vi "solar QTimers Launch.vi"(6 "Suppress Errors? (T)":bool=TRUE, 8 "error in (no error)":errorcluster, 10 "Default QTimers":T1[](array[typedef]), 11 "solar in":refnum<class "solar.lvclass">) -> (0 "error out":errorcluster, 3 "solar out":refnum<class "solar.lvclass">)   [LabVIEW 2018]
doc: "This loads the QTimers from the target's configuration file.\nQTimers = \"TEST1,TEST2\"\nQTimer_TEST1 = \"1000,false,IgnoreIfExists\" # Test 1 QTimer EnQ's every second\nQTimer_TEST1_Msgs = \"READ{bool:true,dbl:3.14}\"\nQTimer_TEST2 = \"5000\" # Test 2 QTimer EnQ's every 5 seconds\nQTimer_TEST2_Msgs = \"READ{bool:true,dbl:3.14}\""
uses:
  qtimer/solar_qtimer_ctl QTimer Settings.ctl
  cfg/solar_cfg Read File (Str).vi
  solar.lvclass
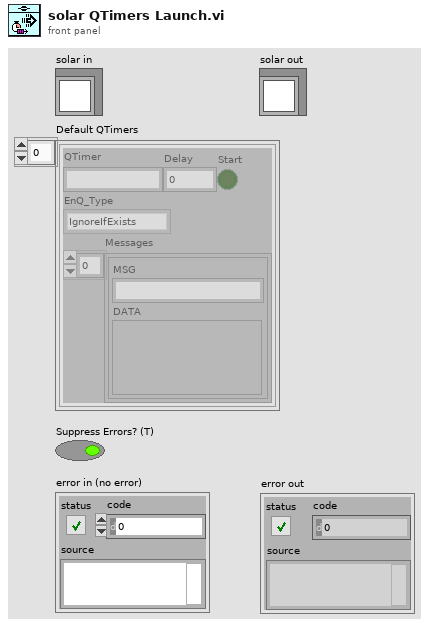
[diagram p1: front panel]
types:
  T1 = typedef "solar_qtimer_ctl QTimer Settings.ctl" = cluster{"QTimer":string, "Delay":i32, "Start":bool, "EnQ_Type":enum8{"Normal", "Priority", "IgnoreIfExists"}, "Messages":cluster{"MSG":string, "DATA":variant}[]}
  T2 = typedef "solar_qtimer_ctl Refnum.ctl" = refnum<k1>
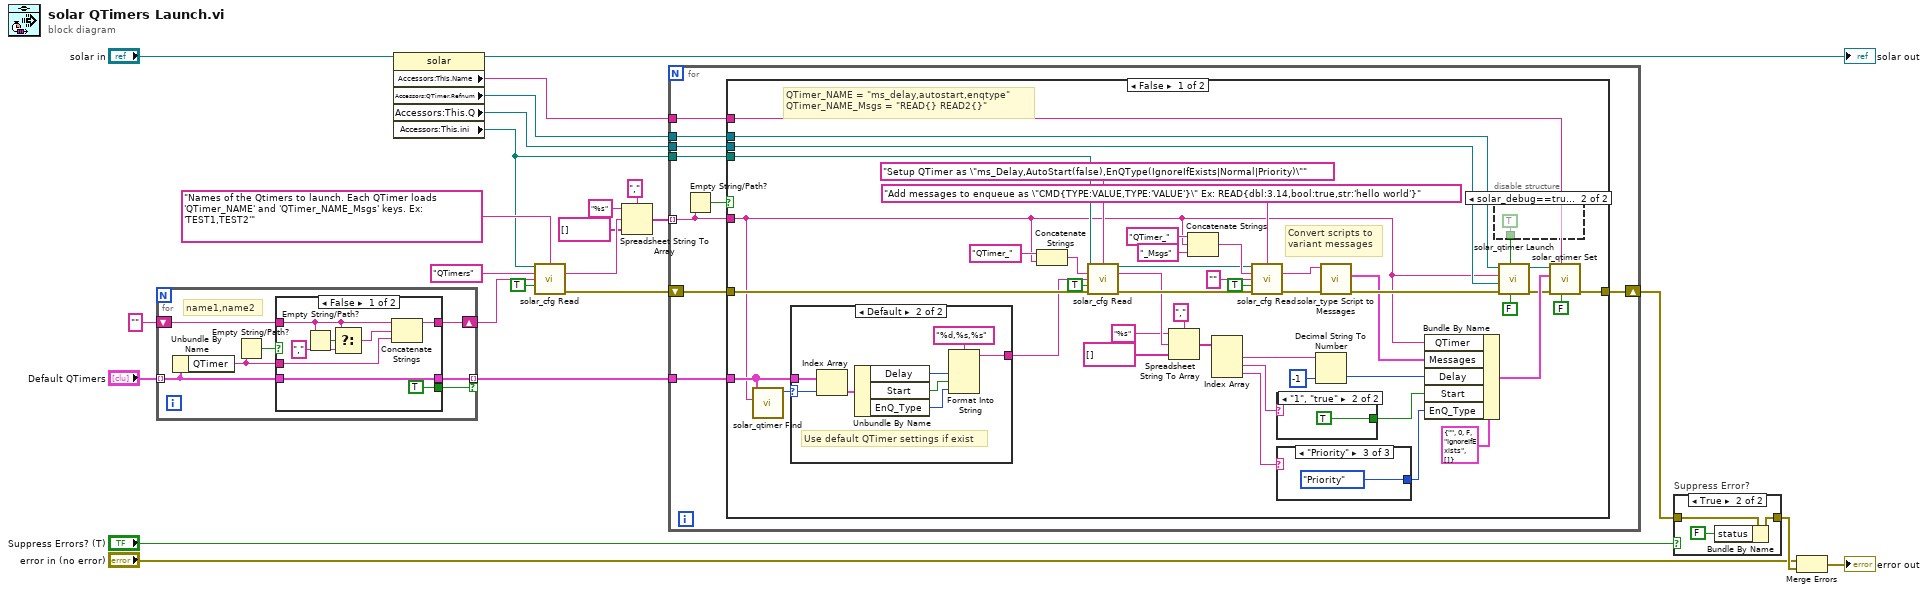
[diagram p0: block diagram]
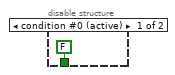
[diagram p2: hidden frame]
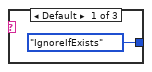
[diagram p3: hidden frame]
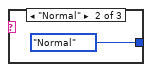
[diagram p4: hidden frame]
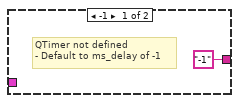
[diagram p6: hidden frame]
diagram:
  n1 = for {
    tunnel: "Default QTimers" -> [w26] mode=indexing
    shift-right: [w29] -> w6
    shift-left: "" -> [w30]
    tunnel: [w27] -> w3 mode=indexing if=w25
    # "name1,name2"
    n2 = Unbundle By Name(w26) -> ("QTimer"=w31:string)
    n3 = Empty String/Path?(string/path=w31) -> (empty?=w28:bool)
    n4 = case shown="False" w28 {
      tunnel: w31 -> [w34 _]
      tunnel: w30 -> [w36 w40]
      tunnel: [w35 w40] -> w29
      tunnel: [w33 _] -> w27
      tunnel: w26 -> [w33 _]
      tunnel: [TRUE _] -> w25
      frame False {
        n5 = Empty String/Path?(string/path=w36) -> (empty?=w39:bool)
        n6 = Select(t=w36, s=w39, f=",") -> (s? t:f=w38:string)
        n7 = Concatenate Strings(w36, w38, w34) -> (w35:string)
      }
      frame True {
      }
    }
  }
  n8 = property class="solar"(reference="solar in") -> (reference out=→"solar out":refnum<class "solar.lvclass">, "Accessors:This.Name"=w1:string, "Accessors:QTimer.Refnum"=w2:T2, "Accessors:This.Q"=w9:refnum<queue>, "Accessors:This.ini"=w4:path)  [unwired: 1 in, 1 out]
  n9 = call-poly "solar_cfg Read.vi"("Config Path (*.ini)"=w4, "Comment"="Names of the Qtimers to launch. Each QTimer loads 'QTimer_NAME' and 'QTimer_NAME_Msgs' keys. Ex: 'TEST1,TEST2'", "Key"="QTimers", "Value in"=w6, "Add Quotes? (T)"=TRUE) -> ("Value out"=w13:string, "error out"=w14:errorcluster)  [unwired: 7 in, 2 out]
  n10 = Spreadsheet String To Array(delimiter (Tab)=",", format string="%s", spreadsheet string=w13, array type (2D Dbl)=string[] []) -> (array=w5:string[])
  n11 = for {
    tunnel: w9 -> [w47]
    tunnel: w2 -> [w46]
    shift-right: [w49] -> w19
    shift-left: w14 -> [w48]
    tunnel: w5 -> [w44] mode=indexing
    tunnel: w4 -> [w43]
    tunnel: w3 -> [w42]
    tunnel: w1 -> [w41]
    n12 = Empty String/Path?(string/path=w44) -> (empty?=w45:bool)
    n13 = case shown="False" w45 {
      tunnel: [w93 w110] -> w49
      tunnel: w48 -> [w87 w110]
      tunnel: w47 -> [w89 _]
      tunnel: w46 -> [w88 _]
      tunnel: w44 -> [w53 _]
      tunnel: w43 -> [w86 _]
      tunnel: w42 -> [w54 _]
      tunnel: w41 -> [w50 _]
      frame False {
        # "QTimer_NAME = \"ms_delay,autostart,enqtype\"\nQTimer_NAME_Msgs = \"READ{} READ2{}\""
        # "Convert scripts to\nvariant messages"
        n14 = call "solar_qtimer Find.vi"("QTimer"=w53, "QTimer Settings"=w54) -> ("Index"=w52:i32)  [unwired: 8 in, 1 out]
        n15 = case shown="Default" w52 {
          selector: w52 -> [_ w108]
          tunnel: w54 -> [_ w109]
          tunnel: ["-1" w102] -> w73
          frame -1 {
            # "QTimer not defined\n- Default to ms_delay of -1"
          }
          frame Default {
            # "Use default QTimer settings if exist"
            n16 = Index Array(array=w109, index=w108) -> (element=w107:T1)
            n17 = Unbundle By Name(w107) -> ("Delay"=w106:i32, "Start"=w105:bool, "EnQ_Type"=w104:enum8{"Normal", "Priority", "IgnoreIfExists"})
            n18 = Format Into String(format string="%d,%s,%s", w106, w105, w104) -> (resulting string=w102:string)  [unwired: 2 in, 1 out]
          }
        }
        n19 = Concatenate Strings("QTimer_" ("Key"), w53) -> (w84:string)
        n20 = call-poly "solar_cfg Read.vi"("Config Path (*.ini)"=w86, "Comment"="Setup QTimer as \"ms_Delay,AutoStart(false),EnQType(IgnoreIfExists|Normal|Priority)\"", "Key"=w84, "Value in"=w73, "Add Quotes? (T)"=TRUE, "error in (no error)"=w87) -> ("Config Path out"=w79:path, "Value out"=w72:string, "error out"=w80:errorcluster)  [unwired: 6 in, 1 out]
        n21 = Spreadsheet String To Array(delimiter (Tab)=",", format string="%s", spreadsheet string=w72, array type (2D Dbl)=string[] []) -> (array=w68:string[])
        n22 = Concatenate Strings("QTimer_" ("Key"), w53, "_Msgs" ("string")) -> (w82:string)
        n23 = Index Array(array=w68) -> (element #1=w67:string, element #2=w61:string, element #3=w59:string)  [unwired: 3 in]
        n24 = call-poly "solar_cfg Read.vi"("Config Path (*.ini)"=w79, "Comment"="Add messages to enqueue as \"CMD{TYPE:VALUE,TYPE:'VALUE'}\" Ex: READ{dbl:3.14,bool:true,str:'hello world'}", "Key"=w82, "Value in"="", "Add Quotes? (T)"=TRUE, "error in (no error)"=w80) -> ("Value out"=w64:string, "error out"=w65:errorcluster)  [unwired: 6 in, 2 out]
        n25 = case shown="\"1\", \"true\"" w61 {
          tunnel: [_ TRUE] -> w60
          frame Default {
          }
          frame "1", "true" {
          }
        }
        n26 = case shown="\"Priority\"" w59 {
          tunnel: [enum8{"Normal", "Priority", "IgnoreIfExists"}."IgnoreIfExists" ("EnQ_Type") enum8{"Normal", "Priority", "IgnoreIfExists"}."Normal" ("EnQ_Type") enum8{"Normal", "Priority", "IgnoreIfExists"}."Priority" ("EnQ_Type")] -> w58
          frame Default {
          }
          frame "Normal" {
          }
          frame "Priority" {
          }
        }
        n27 = Decimal String To Number(string=w67, default (0L)=-1 ("default (0 I32)")) -> (number=w62:i32)  [unwired: 1 in, 1 out]
        n28 = call "solar_type Script to Messages.vi"("error in (no error)"=w65, "Script String"=w64) -> ("error out"=w63:errorcluster, "Messages"=w56:cluster{"MSG":string, "DATA":variant}[])  [unwired: 6 in, 2 out]
        n29 = Bundle By Name(cluster=T1 {"QTimer"="", "Delay"=0, "Start"=FALSE, "EnQ_Type"=enum."IgnoreIfExists", "Messages"=[]} ("Settings"), "QTimer"=w53, "Messages"=w56, "Delay"=w62, "Start"=w60, "EnQ_Type"=w58) -> (w90:T1)
        n30 = disable-structure shown="solar_debug==true" {
          disable-tunnel: [FALSE TRUE ("Open FP? (F)")] -> w51
          frame condition #0 (active) {
          }
          frame condition #1 {
          }
        }
        n31 = call "solar_qtimer Launch.vi"("Suppress Errors? (T)"=FALSE, "Open FP? (F)"=w51, "error in (no error)"=w63, "Target Queue"=w89, "QTimer Name"=w53, "QTimer Refnum in"=w88) -> ("error out"=w57:errorcluster, "QTimer Refnum out"=w55:T2)  [unwired: 4 in]
        n32 = call "solar_qtimer Set.vi"("Suppress Errors? (T)"=FALSE, "Target Name"=w50, "error in (no error)"=w57, "Settings"=w90, "QTimer Refnum in"=w55) -> ("error out"=w93:errorcluster)  [unwired: 5 in, 1 out]
      }
      frame True {
        # "Invalid QTimer name\n- Do nothing"
      }
    }
  }
  n33 = case "Suppress Error?" shown="True" "Suppress Errors? (T)" {
    tunnel: w19 -> [w111 w114]
    tunnel: [w111 w113] -> w23
    frame False {
    }
    frame True {
      n34 = Bundle By Name(cluster=w114, "status"=FALSE) -> (w113:errorcluster)
    }
  }
  n35 = Merge Errors("error in (no error)", w23) -> (→"error out":errorcluster)
